vi "rolling buffer.vi"(7 "mem size":i32=5, 8 "Ch2 2":dbl, 9 "Ch2":dbl, 10 "Ch1":dbl, 11 "current time":timestamp) -> (3 "XY Graph":cluster{timestamp[], dbl[]}[](graph))   [LabVIEW 2019, in "Application.lvclass"]
uses:
  Application.lvclass
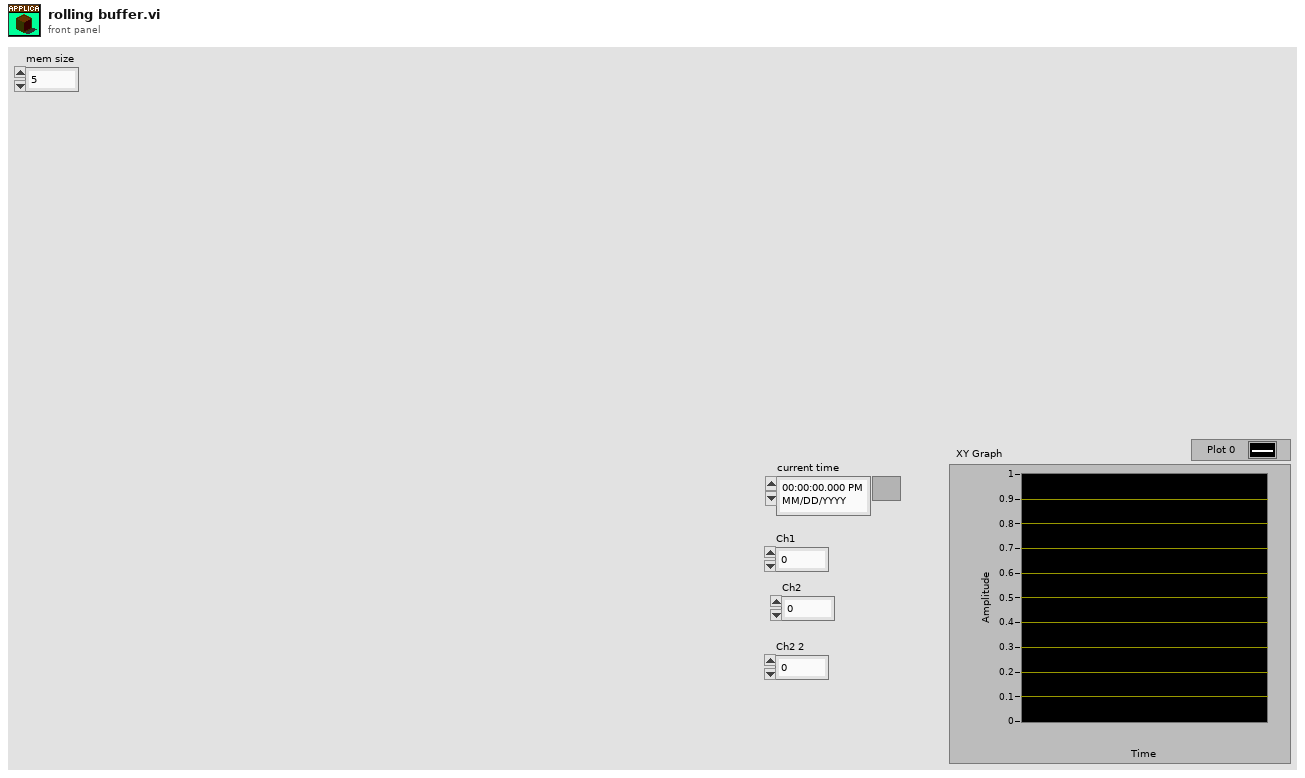
[diagram p1: front panel]
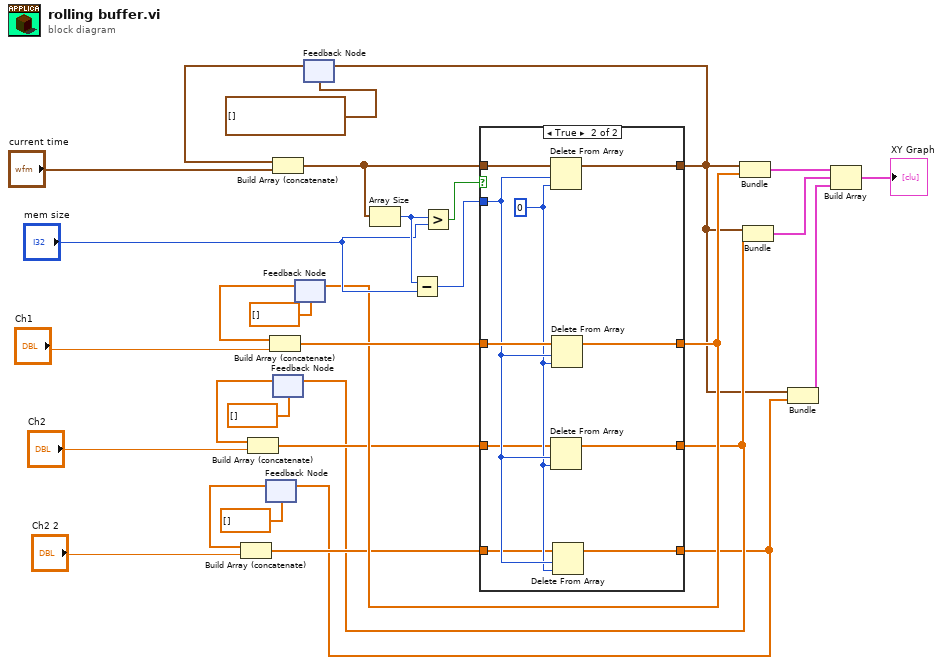
[diagram p0: block diagram]
diagram:
  n1 = feedback #1(dbl[] []) -> (w14:dbl[])
  n2 = Build Array (concatenate)(w14, "Ch2 2") -> (w12:dbl[])
  n3 = feedback #2(dbl[] []) -> (w16:dbl[])
  n4 = Build Array (concatenate)(w16, "Ch2") -> (w15:dbl[])
  n5 = feedback #3(dbl[] []) -> (w24:dbl[])
  n6 = Build Array (concatenate)(w24, "Ch1") -> (w19:dbl[])
  n7 = feedback #4(timestamp[] []) -> (w27:timestamp[])
  n8 = Build Array (concatenate)(w27, "current time") -> (w26:timestamp[])
  n9 = Array Size(array=w26) -> (size(s)=w22:i32)
  n10 = Subtract(x=w22, y="mem size") -> (x-y=w21:i32)
  n11 = Greater?(x=w22, y="mem size") -> (0:w25:bool)
  n12 = case shown="True" w25 {
    tunnel: w26 -> [w32 w42]
    tunnel: [w32 w41] -> w5
    tunnel: w21 -> [_ w38]
    tunnel: w19 -> [w31 w40]
    tunnel: [w31 w39] -> w18
    tunnel: w15 -> [w30 w36]
    tunnel: [w30 w35] -> w11
    tunnel: w12 -> [w29 w34]
    tunnel: [w29 w33] -> w10
    frame False {
    }
    frame True {
      w37 = 0 ("index")
      n13 = Delete From Array(array=w42, length=w38, index=w37) -> (array with subset deleted=w41:timestamp[])  [unwired: 1 out]
      n14 = Delete From Array(array=w36, length=w38, index=w37) -> (array with subset deleted=w35:dbl[])  [unwired: 1 out]
      n15 = Delete From Array(array=w40, length=w38, index=w37) -> (array with subset deleted=w39:dbl[])  [unwired: 1 out]
      n16 = Delete From Array(array=w34, length=w38, index=w37) -> (array with subset deleted=w33:dbl[])  [unwired: 1 out]
    }
  }
  n17 = feedback-in #1(w10) -> ()
  n18 = feedback-in #2(w11) -> ()
  n19 = feedback-in #3(w18) -> ()
  n20 = feedback-in #4(w5) -> ()
  n21 = Bundle(w5, w18) -> (w7:cluster{timestamp[], dbl[]})  [unwired: 1 in]
  n22 = Bundle(w5, w11) -> (w9:cluster{timestamp[], dbl[]})  [unwired: 1 in]
  n23 = Bundle(w5, w10) -> (w8:cluster{timestamp[], dbl[]})  [unwired: 1 in]
  n24 = Build Array(w7, w9, w8) -> (→"XY Graph":cluster{timestamp[], dbl[]}[])
